vi "Sr530 Set Param.vi"(0 "Ressource VISA":refnum<visa-resource-name>="GPIB0::8::INSTR", 1 "Param":T1, 2 "Sensitivity":u16(ring)=1 items=["10 nV"=1, "20 nV"=2, "50 nV"=3, "100 nV"=4, "200 nV"=5, "500 nV"=6, "1 µV"=7, "2 µV"=8, "5 µV"=9, "10 µV"=10, "20 µV"=11, "50 µV"=12, "100µV"=13, "200 µV"=14, "500µV"=15, "1 mV"=16, "2 mV"=17, "5 mV"=18, "10 mV"=19, "20 mV"=20, "50 mV"=21, "100 mV"=22, "200 mV"=23, "500 mV"=24], 3 "Dynamic Res.":u16(ring) items=["Low", "Normal", "High"], 4 "Channels Settings":u16(ring) items=["X, Y", "X Offset, Y Offset", "R, Teta", "R Offset, Teta", "X Noise, Y Noise", "X5 (D/A), X6 (D/A)"], 5 "error in (no error)":errorcluster, 6 "Filters":T2, 7 "Pre Time":u16(ring)=1 items=["1 ms"=1, "3 ms"=2, "10 ms"=3, "30 ms"=4, "100 ms"=5, "300 ms"=6, "1 s"=7, "3 s"=8, "10 s"=9, "30 s"=10, "100 s"=11], 8 "Expand":cluster{"Expand Ch1":bool, "Expand Ch2":bool}, 9 "Post Time":u16(ring) items=["None", "0.1 s", "1 s"]) -> (14 "Ressource VISA Out":refnum<visa-resource-name>="GPIB0::8::INSTR", 19 "error out":errorcluster)   [LabVIEW 2019]
uses:
  <userlib>/SR530/SetParam.ctl
panel:
  in  "Reference Trigger":u16(ring) items=["Positive", "Symmetric", "Negative"]
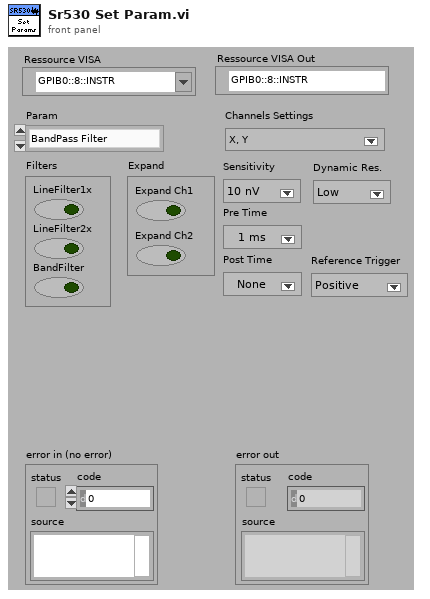
[diagram p1: front panel]
types:
  T1 = typedef "SetParam.ctl" = enum16{"BandPass Filter", "Dynamic Reserve", "Expand", "Ref Trig", "Ch Settings", "Gain", "Notch Filter", "Pre Time Constant", "Post Time Constant"}
  T2 = cluster{"LineFilter1x":bool, "LineFilter2x":bool, "BandFilter":bool}
  T3 = cluster{"BandFilter":bool, "LineFilter1x":bool, "LineFilter2x":bool, "Expand Ch1":bool, "Expand Ch2":bool, "Sensitivity":u16, "Dynamic Reserve":u16, "Pre Time":u16, "Post Time":u16, "Reference Trigger":u16, "Channels Settings":u16, "Frequency":dbl}
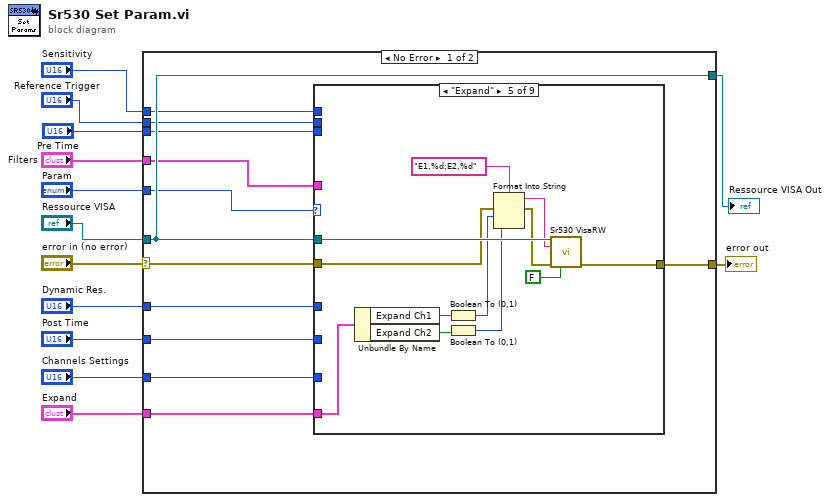
[diagram p0: block diagram]
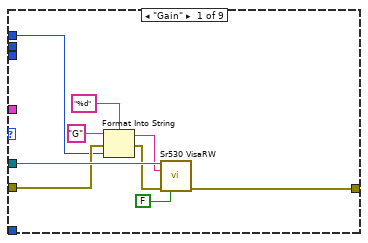
[diagram p2: hidden frame]
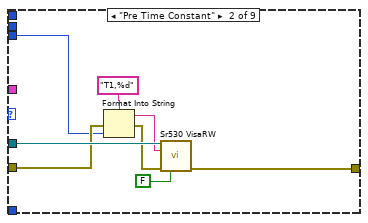
[diagram p3: hidden frame]
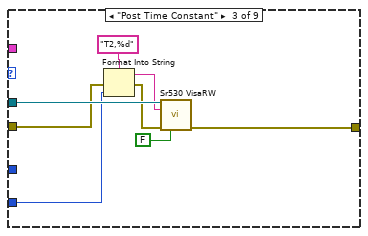
[diagram p4: hidden frame]
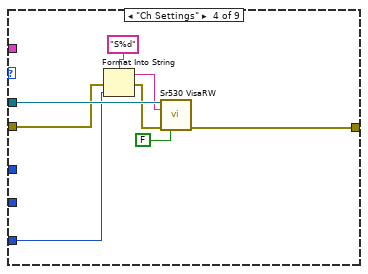
[diagram p5: hidden frame]
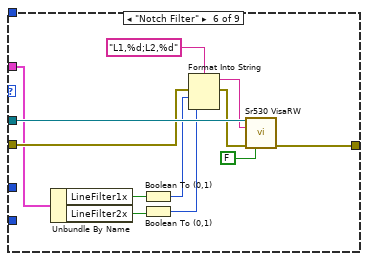
[diagram p6: hidden frame]
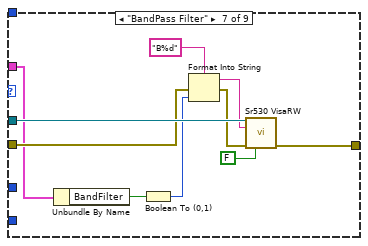
[diagram p7: hidden frame]
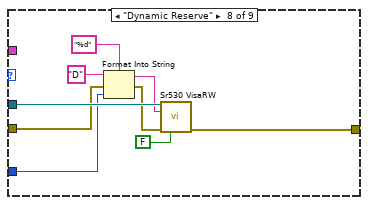
[diagram p8: hidden frame]
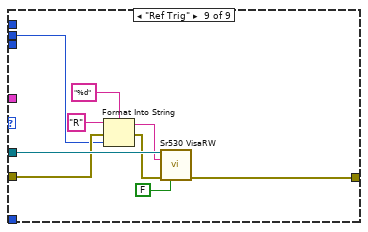
[diagram p9: hidden frame]
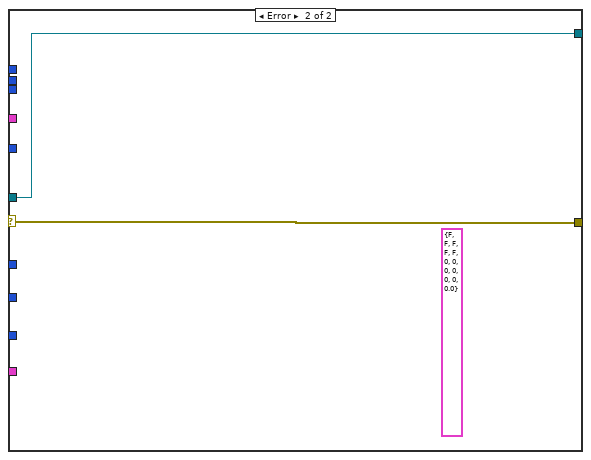
[diagram p10: hidden frame]
diagram:
  n1 = case shown="No Error" "error in (no error)" {
    selector: "error in (no error)" -> [w24 w112]
    tunnel: [w25 w112] -> w12
    tunnel: [w23 w111] -> w11
    tunnel: "Ressource VISA" -> [w23 w111]
    tunnel: "Param" -> [w22 _]
    tunnel: "Filters" -> [w21 _]
    tunnel: "Sensitivity" -> [w20 _]
    tunnel: "Dynamic Res." -> [w19 _]
    tunnel: "Expand" -> [w18 _]
    tunnel: "Pre Time" -> [w17 _]
    tunnel: "Post Time" -> [w16 _]
    tunnel: "Channels Settings" -> [w15 _]
    tunnel: "Reference Trigger" -> [w14 _]
    frame No Error {
      n2 = case shown="\"Expand\"" w22 {
        tunnel: w24 -> [w30 w39 w47 w55 w67 w79 w89 w97 w106]
        tunnel: [w33 w41 w49 w57 w69 w81 w91 w100 w109] -> w25
        tunnel: w23 -> [w34 w42 w50 w58 w70 w82 w92 w101 w110]
        tunnel: w21 -> [_ _ _ _ _ w71 w83 _ _]
        tunnel: w20 -> [w28 _ _ _ _ _ _ _ _]
        tunnel: w19 -> [_ _ _ _ _ _ _ w93 _]
        tunnel: w18 -> [_ _ _ _ w63 _ _ _ _]
        tunnel: w17 -> [_ w35 _ _ _ _ _ _ _]
        tunnel: w16 -> [_ _ w43 _ _ _ _ _ _]
        tunnel: w15 -> [_ _ _ w51 _ _ _ _ _]
        tunnel: w14 -> [_ _ _ _ _ _ _ _ w102]
        frame "Gain" {
          n3 = Format Into String(format string="%d" ("chaîne de format"), initial string="G" ("ChaineCom"), error in=w30, w28) -> (resulting string=w27:string, error out=w29:errorcluster)
          n4 = call <userlib>:"Sr530 VisaRW.vi"("VISA Rsrc"=w34, "ChaineCom"=w27, "error in (no error)"=w29, "Lecture?(T)"=FALSE) -> ("error out"=w33:errorcluster)  [unwired: 6 in, 5 out]
        }
        frame "Pre Time Constant" {
          n5 = Format Into String(format string="T1,%d" ("chaîne de format"), error in=w39, w35) -> (resulting string=w37:string, error out=w38:errorcluster)  [unwired: 1 in]
          n6 = call <userlib>:"Sr530 VisaRW.vi"("VISA Rsrc"=w42, "ChaineCom"=w37, "error in (no error)"=w38, "Lecture?(T)"=FALSE) -> ("error out"=w41:errorcluster)  [unwired: 6 in, 5 out]
        }
        frame "Post Time Constant" {
          n7 = Format Into String(format string="T2,%d" ("chaîne de format"), error in=w47, w43) -> (resulting string=w45:string, error out=w46:errorcluster)  [unwired: 1 in]
          n8 = call <userlib>:"Sr530 VisaRW.vi"("VISA Rsrc"=w50, "ChaineCom"=w45, "error in (no error)"=w46, "Lecture?(T)"=FALSE) -> ("error out"=w49:errorcluster)  [unwired: 6 in, 5 out]
        }
        frame "Ch Settings" {
          n9 = Format Into String(format string="S%d" ("chaîne de format"), error in=w55, w51) -> (resulting string=w53:string, error out=w54:errorcluster)  [unwired: 1 in]
          n10 = call <userlib>:"Sr530 VisaRW.vi"("VISA Rsrc"=w58, "ChaineCom"=w53, "error in (no error)"=w54, "Lecture?(T)"=FALSE) -> ("error out"=w57:errorcluster)  [unwired: 6 in, 5 out]
        }
        frame "Expand" {
          n11 = Unbundle By Name(w63) -> ("Expand Ch1"=w62:bool, "Expand Ch2"=w60:bool)
          n12 = Boolean To (0,1)(Boolean=w62) -> (0, 1=w61:i16)
          n13 = Boolean To (0,1)(Boolean=w60) -> (0, 1=w59:i16)
          n14 = Format Into String(format string="E1,%d;E2,%d" ("chaîne de format"), error in=w67, w61, w59) -> (resulting string=w65:string, error out=w66:errorcluster)  [unwired: 1 in]
          n15 = call <userlib>:"Sr530 VisaRW.vi"("VISA Rsrc"=w70, "ChaineCom"=w65, "error in (no error)"=w66, "Lecture?(T)"=FALSE) -> ("error out"=w69:errorcluster)  [unwired: 6 in, 5 out]
        }
        frame "Notch Filter" {
          n16 = Unbundle By Name(w71) -> ("LineFilter1x"=w75:bool, "LineFilter2x"=w73:bool)
          n17 = Boolean To (0,1)(Boolean=w75) -> (0, 1=w74:i16)
          n18 = Boolean To (0,1)(Boolean=w73) -> (0, 1=w72:i16)
          n19 = Format Into String(format string="L1,%d;L2,%d" ("chaîne de format"), error in=w79, w74, w72) -> (resulting string=w77:string, error out=w78:errorcluster)  [unwired: 1 in]
          n20 = call <userlib>:"Sr530 VisaRW.vi"("VISA Rsrc"=w82, "ChaineCom"=w77, "error in (no error)"=w78, "Lecture?(T)"=FALSE) -> ("error out"=w81:errorcluster)  [unwired: 6 in, 5 out]
        }
        frame "BandPass Filter" {
          n21 = Unbundle By Name(w83) -> ("BandFilter"=w85:bool)
          n22 = Boolean To (0,1)(Boolean=w85) -> (0, 1=w84:i16)
          n23 = Format Into String(format string="B%d" ("chaîne de format"), error in=w89, w84) -> (resulting string=w87:string, error out=w88:errorcluster)  [unwired: 1 in]
          n24 = call <userlib>:"Sr530 VisaRW.vi"("VISA Rsrc"=w92, "ChaineCom"=w87, "error in (no error)"=w88, "Lecture?(T)"=FALSE) -> ("error out"=w91:errorcluster)  [unwired: 6 in, 5 out]
        }
        frame "Dynamic Reserve" {
          n25 = Format Into String(format string="%d" ("chaîne de format"), initial string="D" ("ChaineCom"), error in=w97, w93) -> (resulting string=w95:string, error out=w96:errorcluster)
          n26 = call <userlib>:"Sr530 VisaRW.vi"("VISA Rsrc"=w101, "ChaineCom"=w95, "error in (no error)"=w96, "Lecture?(T)"=FALSE) -> ("error out"=w100:errorcluster)  [unwired: 6 in, 5 out]
        }
        frame "Ref Trig" {
          n27 = Format Into String(format string="%d" ("chaîne de format"), initial string="R" ("ChaineCom"), error in=w106, w102) -> (resulting string=w104:string, error out=w105:errorcluster)
          n28 = call <userlib>:"Sr530 VisaRW.vi"("VISA Rsrc"=w110, "ChaineCom"=w104, "error in (no error)"=w105, "Lecture?(T)"=FALSE) -> ("error out"=w109:errorcluster)  [unwired: 6 in, 5 out]
        }
      }
    }
    frame Error {
      (unwired) T3 {"BandFilter"=FALSE, "LineFilter1x"=FALSE, "LineFilter2x"=FALSE, "Expand Ch1"=FALSE, "Expand Ch2"=FALSE, "Sensitivity"=0, "Dynamic Reserve"=0, "Pre Time"=0, "Post Time"=0, "Reference Trigger"=0, "Channels Settings"=0, "Frequency"=0.0} ("LockInPar")
    }
  }
  "error out" <- w12
  "Ressource VISA Out" <- w11
